vi "sub_Format Rx Data.vi"(1 "Output Packet Array":i32[][](array[numeric])) -> (0 "Received Message":string)   [LabVIEW 2015]
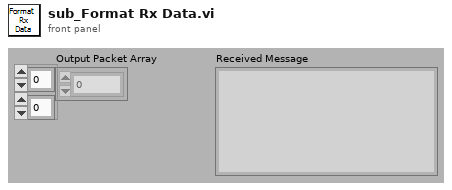
[diagram p1: front panel]
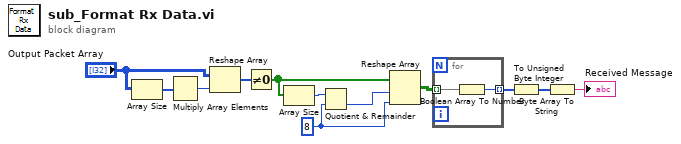
[diagram p0: block diagram]
diagram:
  w8 = 8 ("dimension size")
  n1 = Array Size(array="Output Packet Array") -> (size(s)=w2:i32[])
  n2 = Multiply Array Elements(1:w2) -> (0:w4:i32)
  n3 = Reshape Array("Output Packet Array", w4) -> (w5:i32[])
  n4 = Not Equal To 0?(x=w5) -> (x != 0?=w6:bool[])
  n5 = Array Size(array=w6) -> (size(s)=w7:i32)
  n6 = Quotient & Remainder(x=w7, y=w8) -> (floor(x/y)=w1:i32)  [unwired: 1 out]
  n7 = Reshape Array(w6, w1, w8) -> (w9:bool[][])
  n8 = for {
    tunnel: w9 -> [w14] mode=indexing
    tunnel: [w13] -> w10 mode=indexing
    n9 = Boolean Array To Number(Boolean array=w14) -> (number=w13:u32)
  }
  n10 = To Unsigned Byte Integer(number=w10) -> (unsigned 8bit integer=w11:u8[])
  n11 = Byte Array To String(unsigned byte array=w11) -> (string=→"Received Message":string)
